vi "Autonomous Independent.vi"() -> ()   [LabVIEW 2017]
doc: "This VI is called when autonomous begins, and will automatically be terminated when autonomous ends. You can carry out timed or sensor driven robot movement independently without needing to return to the caller."
uses:
  2017_Steamworks/Programming_Team/Competition/Worlds/Labview/Global 2.vi
  MotionProfiling/FRC_Talon_Motion_Profiles_LV-master/Motion_Profiler_Class/Motion_Profiler_Class-323eb47bd4286328f3a3e236ed86bebf76c73fb1/MotionProfiles.lvclass
  <vilib>/Rock Robotics/Network Tables/NT Write Numeric Array.vi
  <vilib>/Rock Robotics/Network Tables/NT Read Number.vi
  <vilib>/Rock Robotics/Network Tables/NT Read String.vi
panel:
  out "Left Motor":T1(graph)
  out "Right Motor":T1(graph)
  out "Left Throttle":dbl
  out "Left Is Under Run":bool
  out "Left Bottom Buf Count":i32
  out "Right Throttle":dbl
  out "Right Is Under Run":bool
  out "Right Bottom Buf Count":i32
  out "Auto Mode":dbl
  out "Elapsed Time (s) 2":dbl=0.28672027587890625 caption="Elapsed Time (s)"
  out "Time has Elapsed 2":bool=TRUE caption="Time has Elapsed"
  out "Present (s) 2":dbl=3576229234.751028 caption="Present (s)"
  in  "Auton_Modes":T2(array[cluster])=[{"Actions"=[{"Effort"=0.55, "Duration"=3.5, "Action"=enum."Nothing", "Encoder"=0.0, "Condition"=FALSE}, {"Effort"=0.0, "Duration"=0.0, "Action"=enum."Nothing", "Encoder"=0.0, "Condition"=FALSE}]}, {"Actions"=[{"Effort"=0.0, "Duration"=0.1, "Action"=enum."Drive Encoder Reset", "Encoder"=0.0, "Condition"=FALSE}, {"Effort"=0.0, "Duration"=0.1, "Action"=enum."Gyro Reset", "Encoder"=0.0, "Condition"=FALSE}, {"Effort"=0.11, "Duration"=4.0, "Action"=enum."Drive", "Encoder"=72.0, "Condition"=FALSE}, {"Effort"=0.15, "Duration"=0.1, "Action"=enum."Turn", "Encoder"=-55.0, "Condition"=FALSE}, {"Effort"=0.0, "Duration"=0.1, "Action"=enum."Gyro Reset", "Encoder"=0.0, "Condition"=FALSE}, {"Effort"=0.0, "Duration"=0.1, "Action"=enum."Drive Encoder Reset", "Encoder"=0.0, "Condition"=FALSE}, {"Effort"=0.11, "Duration"=4.0, "Action"=enum."Drive", "Encoder"=66.0, "Condition"=FALSE}, {"Effort"=1.0, "Duration"=0.25, "Action"=enum."Gear0", "Encoder"=0.0, "Condition"=FALSE}, {"Effort"=0.0, "Duration"=0.1, "Action"=enum."Drive Encoder Reset", "Encoder"=0.0, "Condition"=FALSE}, {"Effort"=0.11, "Duration"=3.0, "Action"=enum."Drive", "Encoder"=-36.0, "Condition"=TRUE}, {"Effort"=0.08, "Duration"=0.0, "Action"=enum."Turn", "Encoder"=15.5, "Condition"=TRUE}, {"Effort"=0.0, "Duration"=10.0, "Action"=enum."Shoot", "Encoder"=0.0, "Condition"=FALSE}, {"Effort"=0.0, "Duration"=0.5, "Action"=enum."Nothing", "Encoder"=0.0, "Condition"=FALSE}, {"Effort"=0.0, "Duration"=5.0, "Action"=enum."Nothing", "Encoder"=-94.0, "Condition"=TRUE}]}, {"Actions"=[{"Effort"=0.0, "Duration"=0.1, "Action"=enum."Drive Encoder Reset", "Encoder"=0.0, "Condition"=FALSE}, {"Effort"=0.0, "Duration"=0.1, "Action"=enum."Gyro Reset", "Encoder"=0.0, "Condition"=FALSE}, {"Effort"=0.11, "Duration"=4.0, "Action"=enum."Drive", "Encoder"=76.0, "Condition"=FALSE}, {"Effort"=1.0, "Duration"=0.5, "Action"=enum."Gear0", "Encoder"=0.0, "Condition"=FALSE}, {"Effort"=1.0, "Duration"=0.0, "Action"=enum."Nothing", "Encoder"=0.0, "Condition"=FALSE}, {"Effort"=1.0, "Duration"=0.0, "Action"=enum."Nothing", "Encoder"=0.0, "Condition"=FALSE}, {"Effort"=0.0, "Duration"=0.0, "Action"=enum."Drive Encoder Reset", "Encoder"=0.0, "Condition"=FALSE}, {"Effort"=0.0, "Duration"=0.0, "Action"=enum."Nothing", "Encoder"=0.0, "Condition"=FALSE}, {"Effort"=0.0, "Duration"=0.0, "Action"=enum."Nothing", "Encoder"=0.0, "Condition"=FALSE}, {"Effort"=0.0, "Duration"=10000.0, "Action"=enum."Drive", "Encoder"=-24.0, "Condition"=FALSE}, {"Effort"=0.0, "Duration"=0.0, "Action"=enum."Drive Encoder Reset", "Encoder"=0.0, "Condition"=FALSE}, {"Effort"=-0.4, "Duration"=5.0, "Action"=enum."Nothing", "Encoder"=70.0, "Condition"=FALSE}]}, {"Actions"=[{"Effort"=0.0, "Duration"=0.1, "Action"=enum."Drive Encoder Reset", "Encoder"=6.462, "Condition"=FALSE}, {"Effort"=0.0, "Duration"=0.1, "Action"=enum."Gyro Reset", "Encoder"=0.0, "Condition"=FALSE}, {"Effort"=0.0, "Duration"=1.0, "Action"=enum."Drive", "Encoder"=60.0, "Condition"=FALSE}, {"Effort"=0.15, "Duration"=0.1, "Action"=enum."Turn", "Encoder"=55.0, "Condition"=FALSE}, {"Effort"=0.0, "Duration"=0.1, "Action"=enum."Gyro Reset", "Encoder"=0.0, "Condition"=FALSE}, {"Effort"=-0.25, "Duration"=0.0, "Action"=enum."Drive Encoder Reset", "Encoder"=7.5, "Condition"=FALSE}, {"Effort"=0.0, "Duration"=4.0, "Action"=enum."Drive", "Encoder"=76.0, "Condition"=FALSE}, {"Effort"=1.0, "Duration"=0.25, "Action"=enum."Gear0", "Encoder"=0.0, "Condition"=FALSE}, {"Effort"=0.0, "Duration"=0.1, "Action"=enum."Drive Encoder Reset", "Encoder"=0.0, "Condition"=FALSE}, {"Effort"=0.0, "Duration"=3.0, "Action"=enum."Drive", "Encoder"=-36.0, "Condition"=FALSE}, {"Effort"=0.08, "Duration"=0.0, "Action"=enum."Turn", "Encoder"=-60.0, "Condition"=FALSE}, {"Effort"=0.0, "Duration"=0.1, "Action"=enum."Gyro Reset", "Encoder"=0.0, "Condition"=FALSE}, {"Effort"=0.0, "Duration"=0.5, "Action"=enum."Drive Encoder Reset", "Encoder"=0.0, "Condition"=FALSE}, {"Effort"=0.0, "Duration"=5.0, "Action"=enum."Drive", "Encoder"=30.0, "Condition"=TRUE}]}, {"Actions"=[{"Effort"=0.0, "Duration"=0.1, "Action"=enum."Drive Encoder Reset", "Encoder"=6.462, "Condition"=FALSE}, {"Effort"=0.0, "Duration"=0.1, "Action"=enum."Gyro Reset", "Encoder"=0.0, "Condition"=FALSE}, {"Effort"=0.0, "Duration"=1.0, "Action"=enum."Drive", "Encoder"=60.0, "Condition"=FALSE}, {"Effort"=0.15, "Duration"=0.1, "Action"=enum."Turn", "Encoder"=-55.0, "Condition"=FALSE}, {"Effort"=0.0, "Duration"=0.1, "Action"=enum."Gyro Reset", "Encoder"=0.0, "Condition"=FALSE}, {"Effort"=-0.25, "Duration"=0.0, "Action"=enum."Drive Encoder Reset", "Encoder"=7.5, "Condition"=FALSE}, {"Effort"=0.0, "Duration"=4.0, "Action"=enum."Drive", "Encoder"=76.0, "Condition"=FALSE}, {"Effort"=1.0, "Duration"=0.25, "Action"=enum."Gear0", "Encoder"=0.0, "Condition"=FALSE}, {"Effort"=0.0, "Duration"=0.1, "Action"=enum."Drive Encoder Reset", "Encoder"=0.0, "Condition"=FALSE}, {"Effort"=0.0, "Duration"=3.0, "Action"=enum."Drive", "Encoder"=-36.0, "Condition"=FALSE}, {"Effort"=0.08, "Duration"=0.0, "Action"=enum."Turn", "Encoder"=60.0, "Condition"=FALSE}, {"Effort"=0.0, "Duration"=0.1, "Action"=enum."Gyro Reset", "Encoder"=0.0, "Condition"=FALSE}, {"Effort"=0.0, "Duration"=0.5, "Action"=enum."Drive Encoder Reset", "Encoder"=0.0, "Condition"=FALSE}, {"Effort"=0.0, "Duration"=5.0, "Action"=enum."Drive", "Encoder"=30.0, "Condition"=TRUE}]}, {"Actions"=[{"Effort"=0.0, "Duration"=0.1, "Action"=enum."Drive Encoder Reset", "Encoder"=0.0, "Condition"=FALSE}, {"Effort"=0.0, "Duration"=0.1, "Action"=enum."Gyro Reset", "Encoder"=0.0, "Condition"=FALSE}, {"Effort"=0.11, "Duration"=4.0, "Action"=enum."Drive", "Encoder"=72.0, "Condition"=FALSE}, {"Effort"=0.08, "Duration"=0.1, "Action"=enum."Turn", "Encoder"=58.0, "Condition"=FALSE}, {"Effort"=0.0, "Duration"=0.1, "Action"=enum."Gyro Reset", "Encoder"=0.0, "Condition"=FALSE}, {"Effort"=0.0, "Duration"=0.1, "Action"=enum."Drive Encoder Reset", "Encoder"=0.0, "Condition"=FALSE}, {"Effort"=0.11, "Duration"=4.0, "Action"=enum."Drive", "Encoder"=72.0, "Condition"=FALSE}, {"Effort"=1.0, "Duration"=0.25, "Action"=enum."Gear0", "Encoder"=0.0, "Condition"=FALSE}, {"Effort"=0.0, "Duration"=0.1, "Action"=enum."Drive Encoder Reset", "Encoder"=3.0, "Condition"=FALSE}, {"Effort"=0.11, "Duration"=3.0, "Action"=enum."Drive", "Encoder"=-36.0, "Condition"=FALSE}, {"Effort"=0.08, "Duration"=0.0, "Action"=enum."Turn", "Encoder"=-15.5, "Condition"=FALSE}, {"Effort"=0.0, "Duration"=10.0, "Action"=enum."Nothing", "Encoder"=0.0, "Condition"=FALSE}, {"Effort"=0.0, "Duration"=0.5, "Action"=enum."Nothing", "Encoder"=0.0, "Condition"=FALSE}, {"Effort"=0.11, "Duration"=0.0, "Action"=enum."Nothing", "Encoder"=-94.0, "Condition"=FALSE}, {"Effort"=0.0, "Duration"=10.0, "Action"=enum."Nothing", "Encoder"=0.0, "Condition"=FALSE}]}, {"Actions"=[{"Effort"=0.0, "Duration"=0.1, "Action"=enum."Drive Encoder Reset", "Encoder"=0.0, "Condition"=FALSE}, {"Effort"=0.0, "Duration"=0.1, "Action"=enum."Gyro Reset", "Encoder"=0.0, "Condition"=FALSE}, {"Effort"=0.2, "Duration"=5.0, "Action"=enum."Drive", "Encoder"=110.0, "Condition"=FALSE}, {"Effort"=0.75, "Duration"=1.0, "Action"=enum."Nothing", "Encoder"=0.0, "Condition"=FALSE}, {"Effort"=0.0, "Duration"=1.0, "Action"=enum."Nothing", "Encoder"=0.0, "Condition"=FALSE}, {"Effort"=0.0, "Duration"=0.0, "Action"=enum."Nothing", "Encoder"=0.0, "Condition"=FALSE}]}, {"Actions"=[{"Effort"=0.0, "Duration"=0.1, "Action"=enum."Drive Encoder Reset", "Encoder"=0.0, "Condition"=FALSE}, {"Effort"=0.0, "Duration"=0.1, "Action"=enum."Gyro Reset", "Encoder"=0.0, "Condition"=FALSE}, {"Effort"=0.3, "Duration"=0.0, "Action"=enum."Drive", "Encoder"=24.0, "Condition"=FALSE}, {"Effort"=0.3, "Duration"=3.0, "Action"=enum."Nothing", "Encoder"=0.0, "Condition"=FALSE}, {"Effort"=0.3, "Duration"=2.0, "Action"=enum."Vision Correction", "Encoder"=30.0, "Condition"=FALSE}, {"Effort"=0.2, "Duration"=1.0, "Action"=enum."Drive", "Encoder"=18.5, "Condition"=TRUE}, {"Effort"=1.0, "Duration"=0.0, "Action"=enum."Gear0", "Encoder"=0.0, "Condition"=FALSE}, {"Effort"=-0.2, "Duration"=1.3, "Action"=enum."Drive", "Encoder"=30.0, "Condition"=TRUE}, {"Effort"=0.0, "Duration"=3.0, "Action"=enum."Nothing", "Encoder"=0.0, "Condition"=FALSE}, {"Effort"=0.03, "Duration"=0.0, "Action"=enum."Turn", "Encoder"=0.0, "Condition"=FALSE}, {"Effort"=0.0, "Duration"=0.0, "Action"=enum."Drive", "Encoder"=0.0, "Condition"=FALSE}]}, {"Actions"=[{"Effort"=0.0, "Duration"=0.0, "Action"=enum."Nothing", "Encoder"=0.0, "Condition"=FALSE}]}, {"Actions"=[{"Effort"=0.0, "Duration"=2.5, "Action"=enum."Shoot", "Encoder"=0.0, "Condition"=FALSE}, {"Effort"=0.0, "Duration"=5.0, "Action"=enum."Index", "Encoder"=0.0, "Condition"=FALSE}, {"Effort"=0.25, "Duration"=3.5, "Action"=enum."Nothing", "Encoder"=88.0, "Condition"=FALSE}, {"Effort"=1.0, "Duration"=1.0, "Action"=enum."Nothing", "Encoder"=0.0, "Condition"=FALSE}, {"Effort"=1.0, "Duration"=1.0, "Action"=enum."Nothing", "Encoder"=0.0, "Condition"=FALSE}, {"Effort"=1.0, "Duration"=0.5, "Action"=enum."Nothing", "Encoder"=0.0, "Condition"=FALSE}, {"Effort"=0.0, "Duration"=0.0, "Action"=enum."Nothing", "Encoder"=0.0, "Condition"=FALSE}, {"Effort"=-0.25, "Duration"=0.0, "Action"=enum."Nothing", "Encoder"=3.0, "Condition"=FALSE}, {"Effort"=0.0, "Duration"=0.0, "Action"=enum."Nothing", "Encoder"=0.0, "Condition"=FALSE}, {"Effort"=0.25, "Duration"=0.0, "Action"=enum."Nothing", "Encoder"=24.0, "Condition"=FALSE}, {"Effort"=0.0, "Duration"=0.0, "Action"=enum."Nothing", "Encoder"=0.0, "Condition"=FALSE}, {"Effort"=-0.25, "Duration"=0.0, "Action"=enum."Nothing", "Encoder"=12.0, "Condition"=FALSE}]}, {"Actions"=[{"Effort"=0.0, "Duration"=0.1, "Action"=enum."Drive Encoder Reset", "Encoder"=0.0, "Condition"=FALSE}, {"Effort"=0.0, "Duration"=1.0, "Action"=enum."Gyro Reset", "Encoder"=0.0, "Condition"=FALSE}, {"Effort"=0.3, "Duration"=1.4, "Action"=enum."Drive", "Encoder"=88.0, "Condition"=FALSE}, {"Effort"=0.3, "Duration"=3.0, "Action"=enum."Turn", "Encoder"=2.0, "Condition"=FALSE}, {"Effort"=1.0, "Duration"=1.0, "Action"=enum."Nothing", "Encoder"=0.0, "Condition"=FALSE}, {"Effort"=1.0, "Duration"=1.0, "Action"=enum."Nothing", "Encoder"=0.0, "Condition"=FALSE}, {"Effort"=0.0, "Duration"=0.0, "Action"=enum."Nothing", "Encoder"=0.0, "Condition"=FALSE}, {"Effort"=-0.25, "Duration"=0.0, "Action"=enum."Nothing", "Encoder"=3.0, "Condition"=FALSE}, {"Effort"=0.0, "Duration"=0.0, "Action"=enum."Nothing", "Encoder"=0.0, "Condition"=FALSE}, {"Effort"=0.25, "Duration"=0.0, "Action"=enum."Nothing", "Encoder"=24.0, "Condition"=FALSE}, {"Effort"=0.0, "Duration"=0.0, "Action"=enum."Nothing", "Encoder"=0.0, "Condition"=FALSE}, {"Effort"=-0.25, "Duration"=0.0, "Action"=enum."Nothing", "Encoder"=12.0, "Condition"=FALSE}]}, {"Actions"=[{"Effort"=0.0, "Duration"=1.0, "Action"=enum."Drive Encoder Reset", "Encoder"=0.0, "Condition"=FALSE}, {"Effort"=0.0, "Duration"=1.0, "Action"=enum."Shoot", "Encoder"=0.0, "Condition"=FALSE}, {"Effort"=0.25, "Duration"=5.0, "Action"=enum."Index", "Encoder"=88.0, "Condition"=FALSE}, {"Effort"=1.0, "Duration"=1.0, "Action"=enum."Nothing", "Encoder"=0.0, "Condition"=FALSE}, {"Effort"=1.0, "Duration"=1.0, "Action"=enum."Nothing", "Encoder"=0.0, "Condition"=FALSE}, {"Effort"=1.0, "Duration"=0.5, "Action"=enum."Nothing", "Encoder"=0.0, "Condition"=FALSE}, {"Effort"=0.0, "Duration"=0.0, "Action"=enum."Nothing", "Encoder"=0.0, "Condition"=FALSE}, {"Effort"=-0.25, "Duration"=0.0, "Action"=enum."Nothing", "Encoder"=3.0, "Condition"=FALSE}, {"Effort"=0.0, "Duration"=0.0, "Action"=enum."Nothing", "Encoder"=0.0, "Condition"=FALSE}, {"Effort"=0.25, "Duration"=0.0, "Action"=enum."Nothing", "Encoder"=24.0, "Condition"=FALSE}, {"Effort"=0.0, "Duration"=0.0, "Action"=enum."Nothing", "Encoder"=0.0, "Condition"=FALSE}, {"Effort"=-0.25, "Duration"=0.0, "Action"=enum."Nothing", "Encoder"=12.0, "Condition"=FALSE}]}, {"Actions"=[{"Effort"=0.0, "Duration"=0.1, "Action"=enum."Drive Encoder Reset", "Encoder"=0.0, "Condition"=FALSE}, {"Effort"=0.0, "Duration"=1.0, "Action"=enum."Gyro Reset", "Encoder"=0.0, "Condition"=FALSE}, {"Effort"=0.0, "Duration"=20.0, "Action"=enum."Drive", "Encoder"=60.0, "Condition"=FALSE}, {"Effort"=0.3, "Duration"=4.0, "Action"=enum."Nothing", "Encoder"=0.0, "Condition"=FALSE}, {"Effort"=1.0, "Duration"=1.0, "Action"=enum."Nothing", "Encoder"=0.0, "Condition"=FALSE}, {"Effort"=1.0, "Duration"=0.5, "Action"=enum."Nothing", "Encoder"=0.0, "Condition"=FALSE}, {"Effort"=0.0, "Duration"=0.0, "Action"=enum."Nothing", "Encoder"=0.0, "Condition"=FALSE}, {"Effort"=0.3, "Duration"=0.5, "Action"=enum."Nothing", "Encoder"=24.0, "Condition"=TRUE}, {"Effort"=0.0, "Duration"=0.0, "Action"=enum."Nothing", "Encoder"=0.0, "Condition"=FALSE}, {"Effort"=-0.2, "Duration"=2.0, "Action"=enum."Nothing", "Encoder"=24.0, "Condition"=TRUE}, {"Effort"=0.0, "Duration"=0.0, "Action"=enum."Nothing", "Encoder"=0.0, "Condition"=FALSE}, {"Effort"=-0.25, "Duration"=0.0, "Action"=enum."Nothing", "Encoder"=12.0, "Condition"=FALSE}]}, {"Actions"=[{"Effort"=0.0, "Duration"=0.1, "Action"=enum."Drive Encoder Reset", "Encoder"=0.0, "Condition"=FALSE}, {"Effort"=0.0, "Duration"=0.1, "Action"=enum."Gyro Reset", "Encoder"=0.0, "Condition"=FALSE}, {"Effort"=0.0, "Duration"=4.0, "Action"=enum."Nothing", "Encoder"=4.0, "Condition"=FALSE}, {"Effort"=0.3, "Duration"=0.1, "Action"=enum."Vision Correction", "Encoder"=24.0, "Condition"=FALSE}, {"Effort"=0.0, "Duration"=0.1, "Action"=enum."Nothing", "Encoder"=0.0, "Condition"=FALSE}, {"Effort"=0.3, "Duration"=4.0, "Action"=enum."Nothing", "Encoder"=68.17, "Condition"=FALSE}, {"Effort"=1.0, "Duration"=0.25, "Action"=enum."Nothing", "Encoder"=0.0, "Condition"=FALSE}, {"Effort"=0.0, "Duration"=0.0, "Action"=enum."Nothing", "Encoder"=3.0, "Condition"=FALSE}, {"Effort"=-0.3, "Duration"=3.0, "Action"=enum."Nothing", "Encoder"=36.0, "Condition"=FALSE}, {"Effort"=0.15, "Duration"=0.0, "Action"=enum."Nothing", "Encoder"=31.5, "Condition"=FALSE}, {"Effort"=0.0, "Duration"=0.1, "Action"=enum."Nothing", "Encoder"=0.0, "Condition"=FALSE}]}]
  # "Be sure to right-click and choose Data Operations>>Make Current Value default if you want to save the array values with the VI"
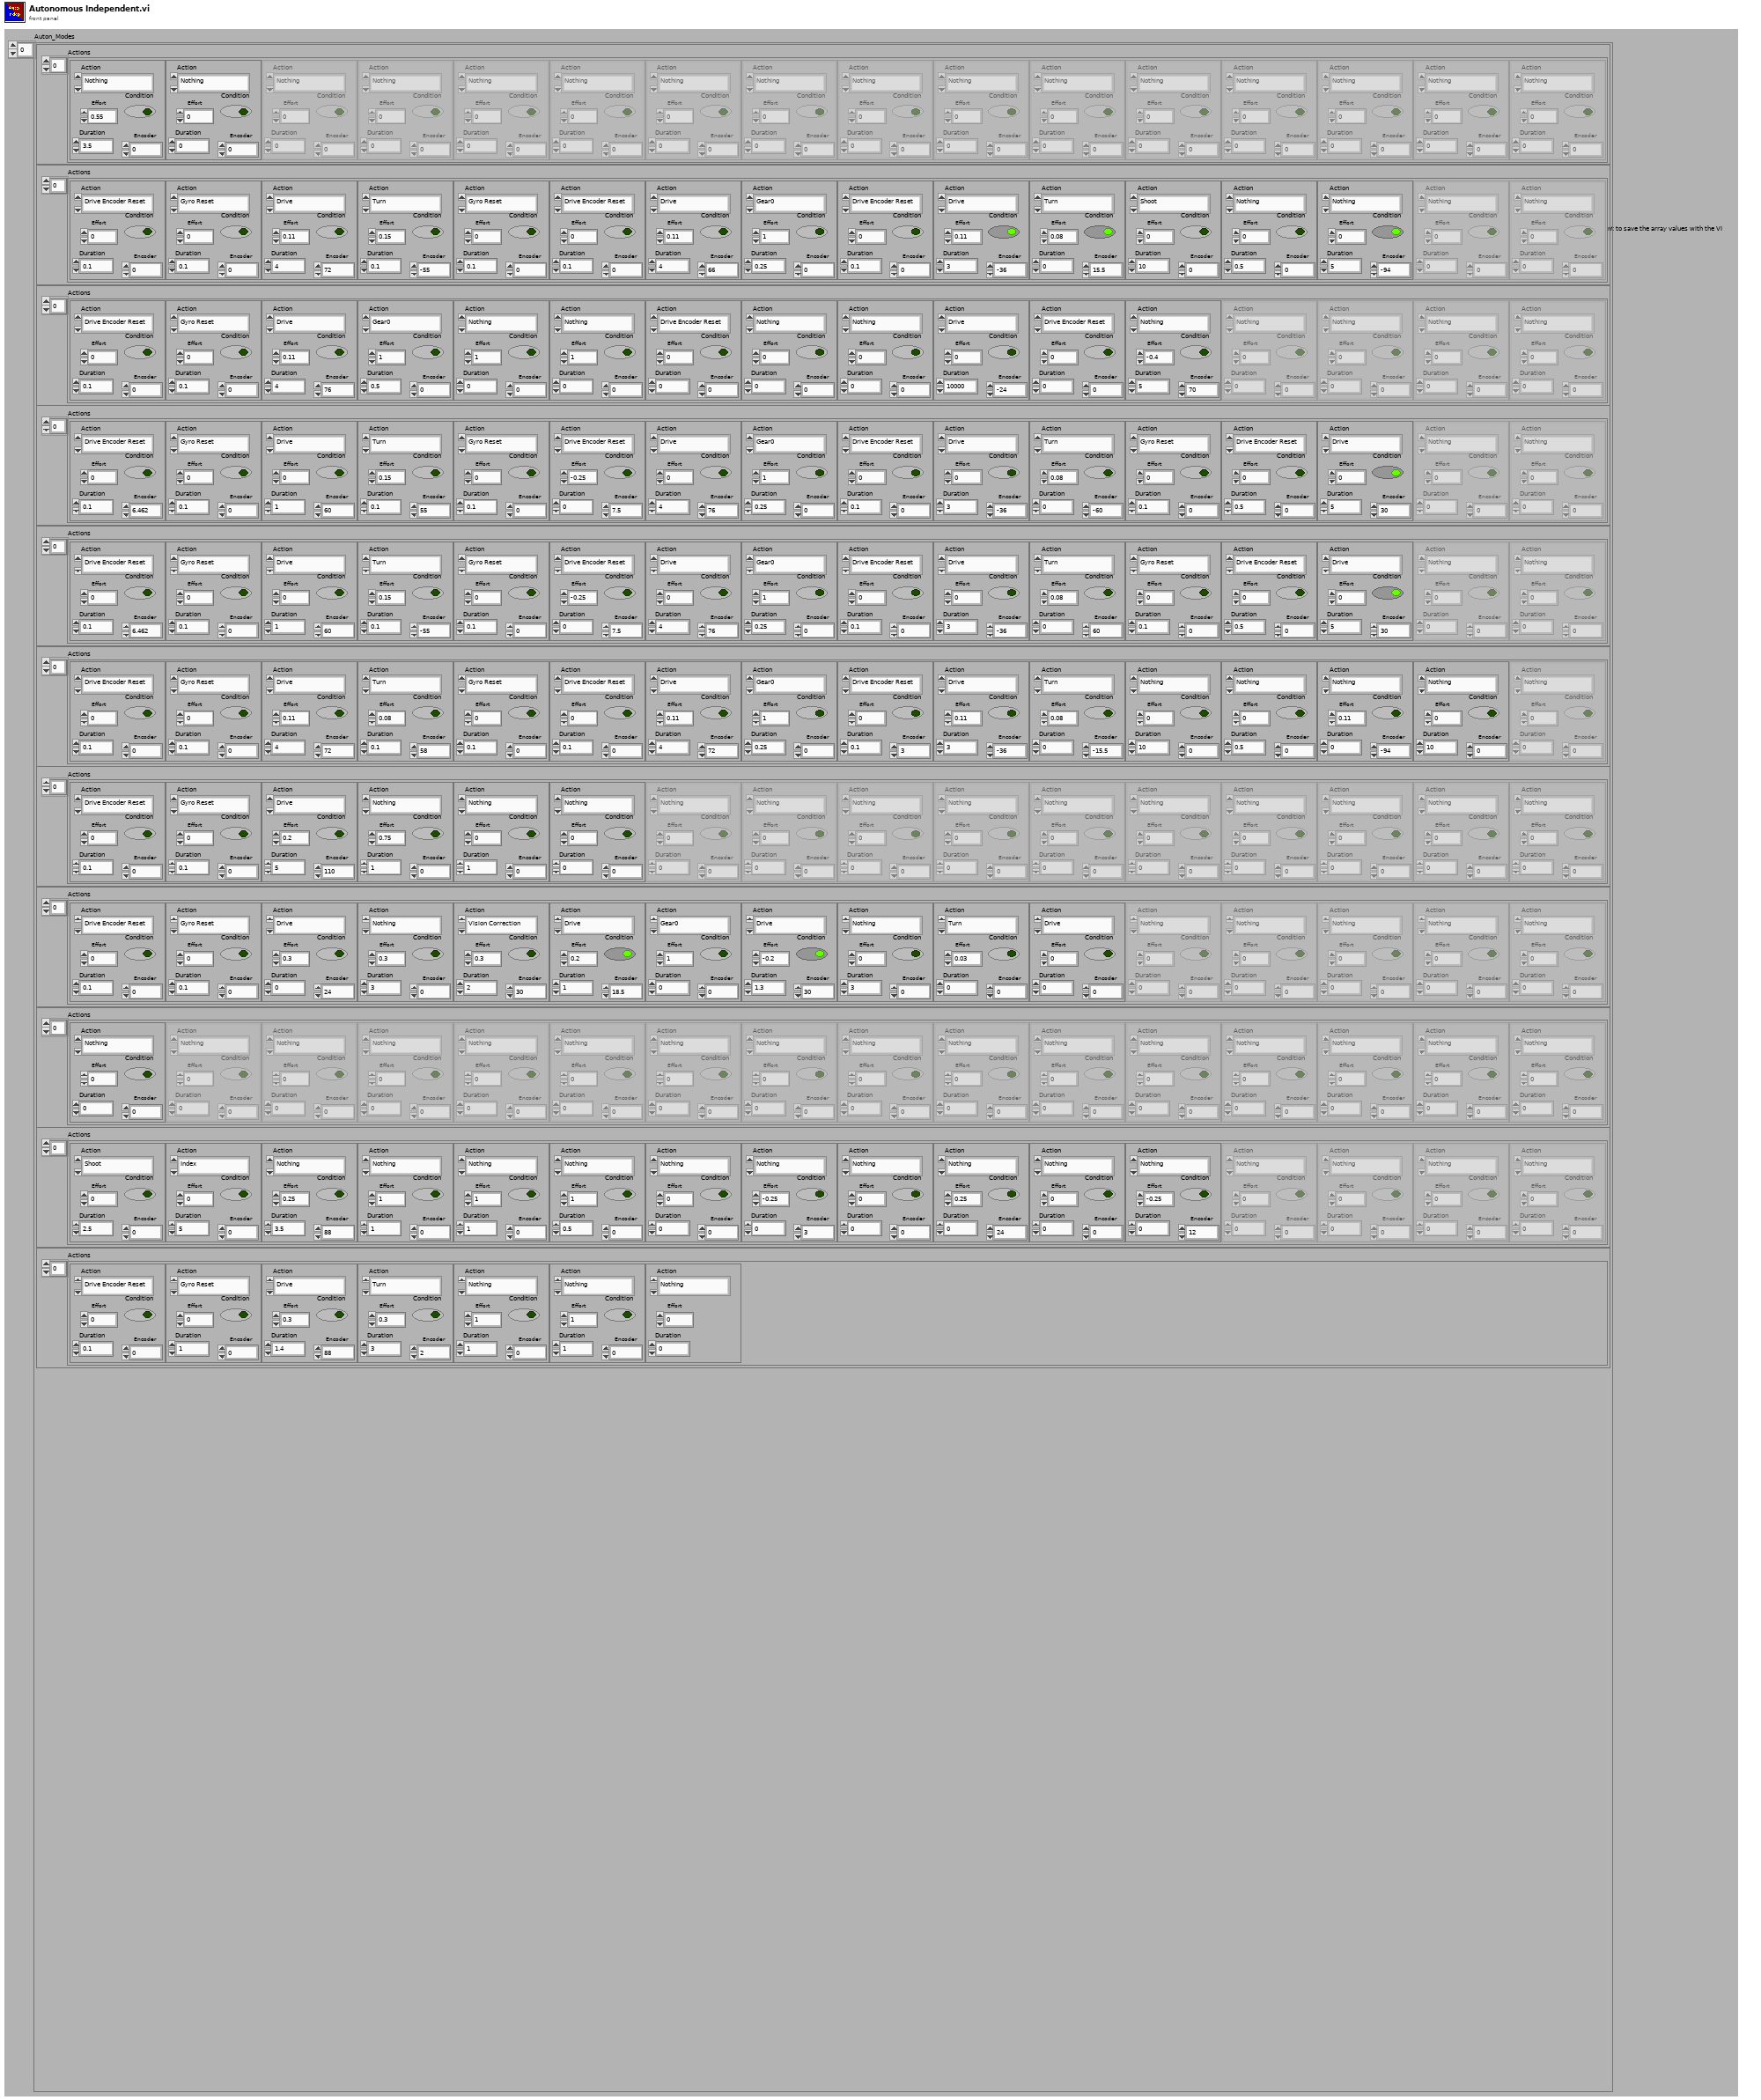
[diagram p1: front panel]
types:
  T1 = cluster{"Set_Vel_(u/100ms)":i32, "Act_Vel_(u/100ms)":i32, "Set_Pos_(u)":i32, "Act_Pos(u)":i32}
  T2 = cluster{"Actions":cluster{"Effort":dbl, "Duration":dbl, "Action":enum16{"Nothing", "Drive", "Vision Correction", "Turn", "Gear0", "Gear1", "Climb", "Intake", "Index", "Shoot", "Test", "Drive Encoder Reset", "Gyro Reset"}, "Encoder":dbl, "Condition":bool}[]}[]
  T3 = typedef "WPI_JoystickDevRef.ctl" = cluster{"Device":T4}
  T4 = typedef "WPI_JoystickDeviceEnum.ctl" = enum16{"USB 0", "USB 1", "USB 2", "USB 3", "USB 4", "USB 5"}
  T5 = cluster{"Actions":cluster{"Effort":dbl, "Duration":dbl, "Action":enum16{"Nothing", "Drive", "Vision Correction", "Turn", "Gear0", "Gear1", "Climb", "Intake", "Index", "Shoot", "Test", "Drive Encoder Reset", "Gyro Reset"}, "Encoder":dbl, "Condition":bool}[]}
  T6 = cluster{"Effort":dbl, "Duration":dbl, "Action":enum16{"Nothing", "Drive", "Vision Correction", "Turn", "Gear0", "Gear1", "Climb", "Intake", "Index", "Shoot", "Test", "Drive Encoder Reset", "Gyro Reset"}, "Encoder":dbl, "Condition":bool}[]
  T7 = typedef "WPI_MotorControlDeviceRef.ctl" = cluster{"DeviceStatus":errorcluster, "Type":T8, "PWM":cluster{"PWM Channel":T9, "DeadBand":T10}, "CAN":cluster{"Device Number":u8, "SetOutput VI Ref":variant, "GetOutput VI Ref":variant, "Enable VI Ref":variant, "Disable VI Ref":variant, "Data":variant}, "Invert":bool, "DIO PWM":cluster{"PWM \"Enable\" Channel":T9, "DIOChannel":T11, "PWM Rate":dbl}}
  T8 = typedef "WPI_MotorControlType.ctl" = enum16{"PWM", "CAN", "DIO PWM"}
  T9 = typedef "FPGA_DIOPWMChannel.ctl" = enum8{"PWM 0", "PWM 1", "PWM 2", "PWM 3", "PWM 4", "PWM 5", "PWM 6", "PWM 7", "PWM 8", "PWM 9", "PWM MXP 0", "PWM MXP 1", "PWM MXP 2", "PWM MXP 3", "PWM MXP 4", "PWM MXP 5", "PWM MXP 6", "PWM MXP 7", "PWM MXP 8", "PWM MXP 9", "Invalid"}
  T10 = typedef "WPI_PWMDeadband.ctl" = cluster{"Name":string, "maxPositivePwm":i32, "minPositivePwm":i32, "centerPwm":i32, "maxNegativePwm":i32, "minNegativePwm":i32, "angularRange":u16}
  T11 = typedef "FPGA_DIOChannel.ctl" = enum8{"DIO 0", "DIO 1", "DIO 2", "DIO 3", "DIO 4", "DIO 5", "DIO 6", "DIO 7", "DIO 8", "DIO 9", "DIO MXP 0", "DIO MXP 1", "DIO MXP 2", "DIO MXP 3", "DIO MXP 4", "DIO MXP 5", "DIO MXP 6", "DIO MXP 7", "DIO MXP 8", "DIO MXP 9", "DIO MXP 10", "DIO MXP 11", "DIO MXP 12", "DIO MXP 13", "DIO MXP 14", "DIO MXP 15", "SPI Port CS1", "SPI Port CS2", "SPI Port CS3", "SPI Port MISO", "SPI Port MOSI", "Invalid"}
  T12 = enum16{"Nothing", "Drive", "Vision Correction", "Turn", "Gear0", "Gear1", "Climb", "Intake", "Index", "Shoot", "Test", "Drive Encoder Reset", "Gyro Reset"}
  T13 = typedef "MotionProfiles.lvclass/MotionProfile_MP_Class_Status.ctl" = cluster{"Motion Profile Status":cluster{"Top Buffer Remaining":i32, "Top Buffer Count":i32, "Bottom Buffer Count":i32, "Has Underrun?":bool, "Is Underrun?":bool, "Active Point Valid?":bool, "Is Last?":bool, "Profile Slot Select 0":i32, "Output Enable":i32, "Time Duration (ms)":i32, "Profile Slot Select 1":i32}, "TalonState":T14, "MP Is Done":bool, "MP Is Executing":bool, "Set_Vel_(u/100ms)":i32, "Set_Pos_(u)":i32, "Act_Vel_(u/100ms)":i32, "Act_Pos(u)":i32, "Throtle":dbl}
  T14 = typedef "MotionProfiles.lvclass/MotionProfile_TalonSetValueEnum.ctl" = enum16{"Disable", "Enable", "Hold"}
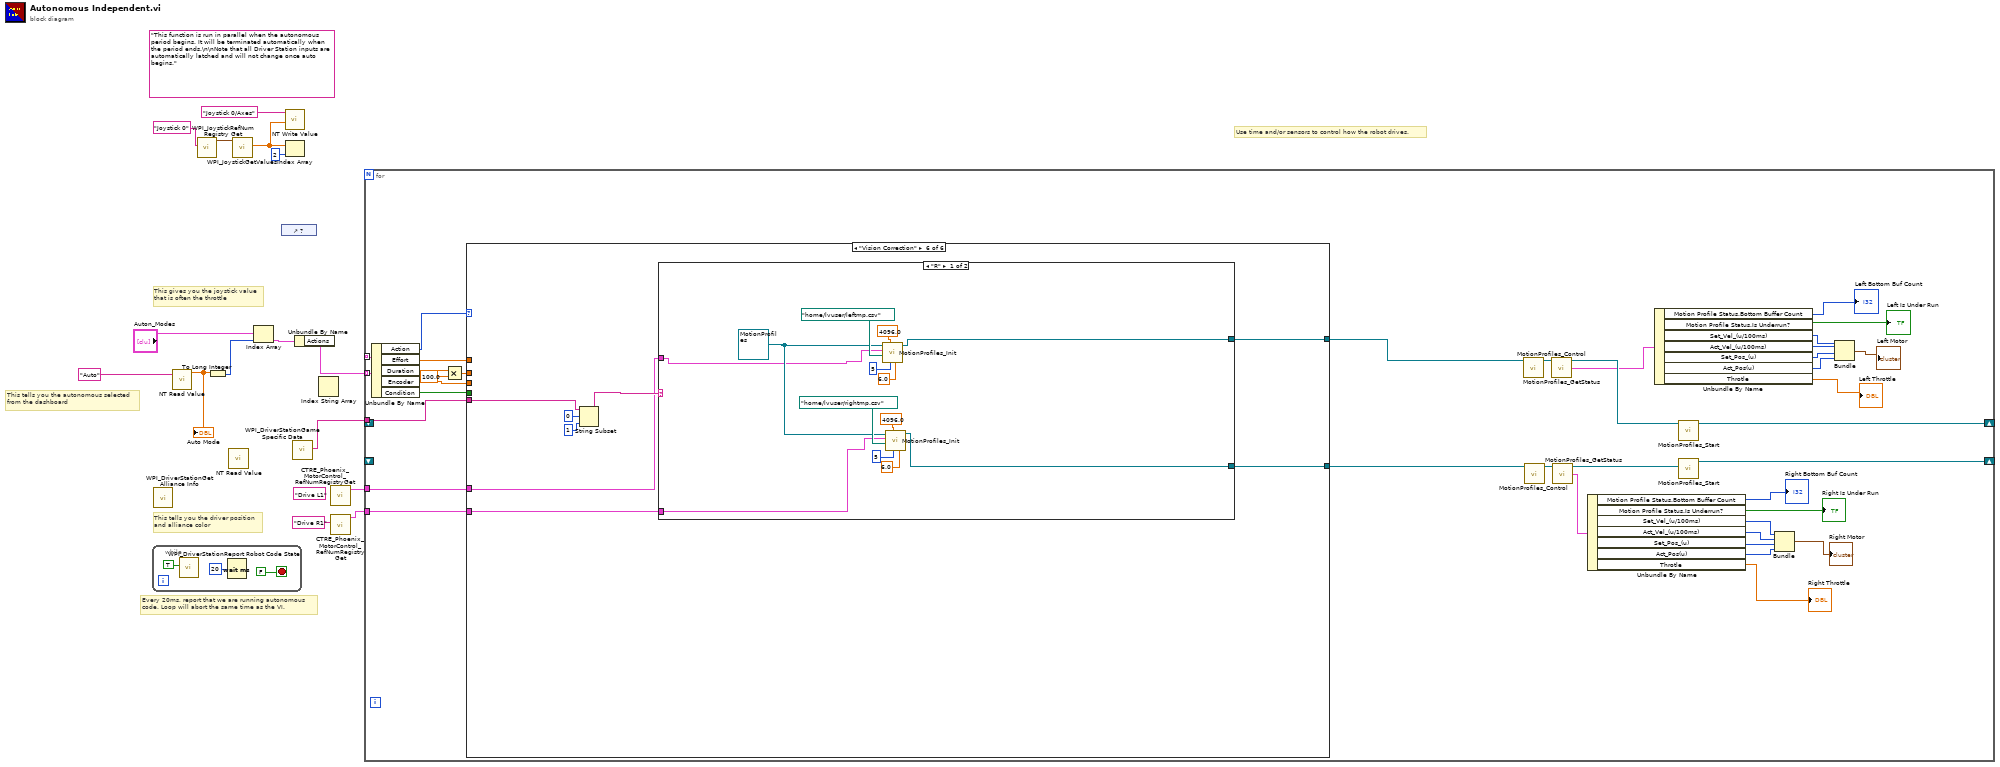
[diagram p0: block diagram]
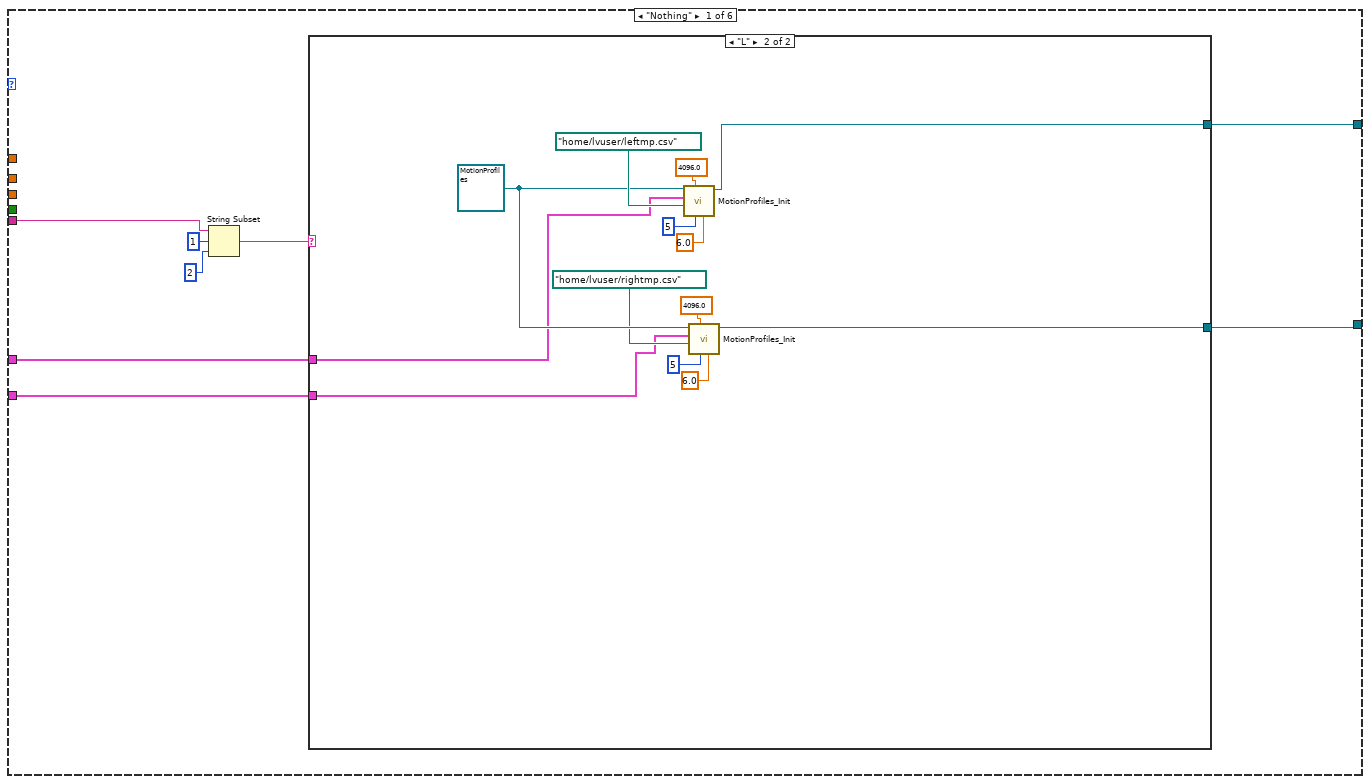
[diagram p2: hidden frame]
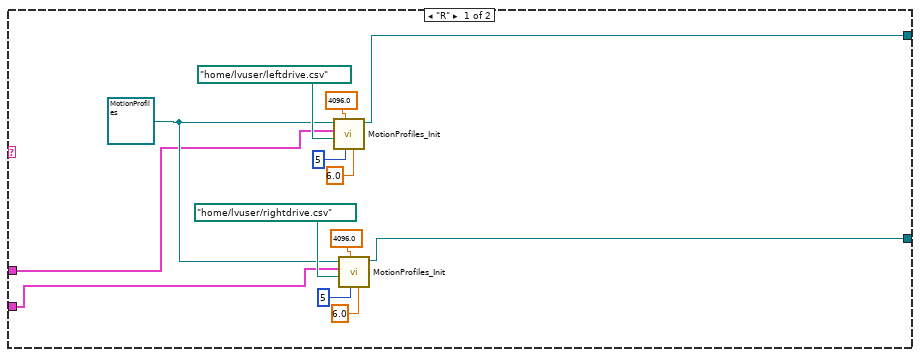
[diagram p3: hidden frame]
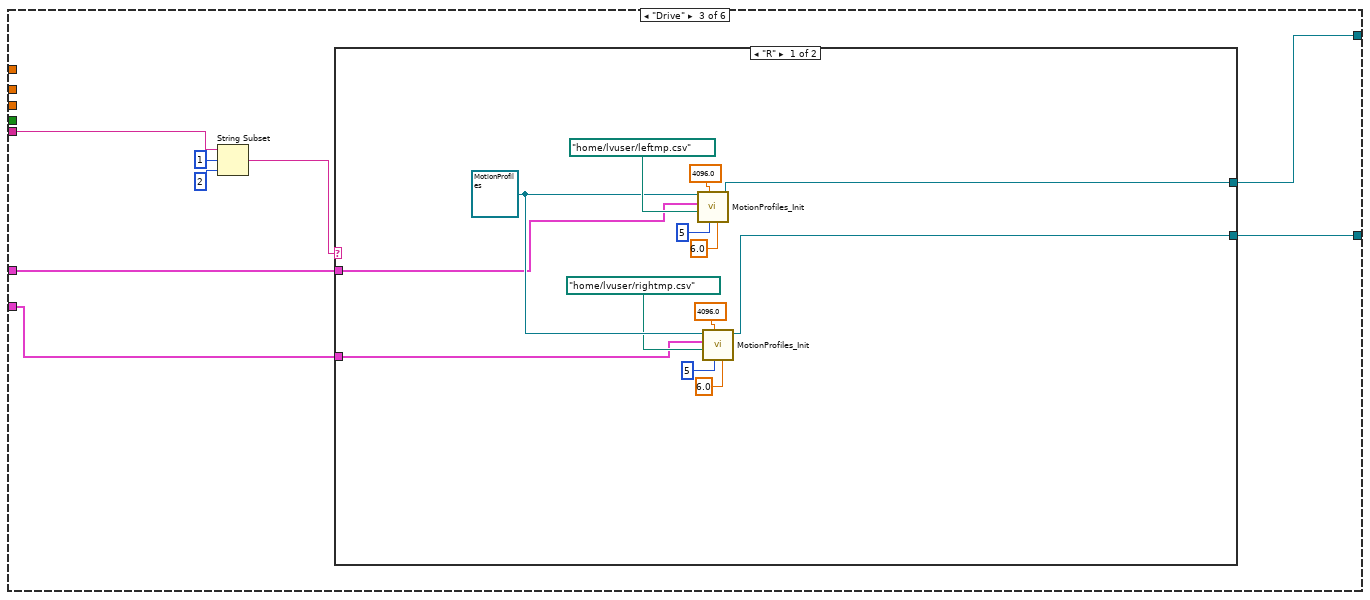
[diagram p5: hidden frame]
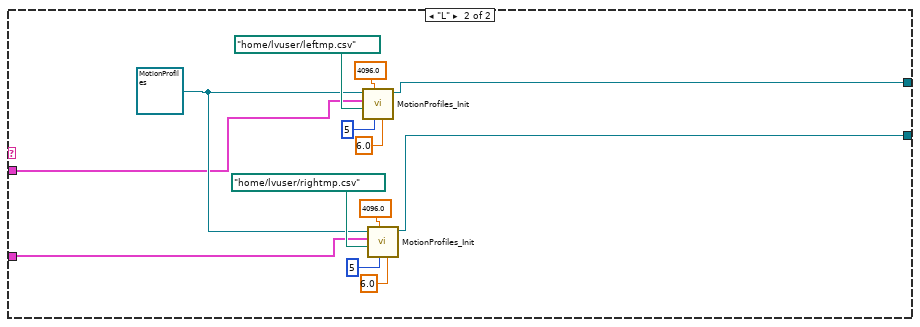
[diagram p6: hidden frame]
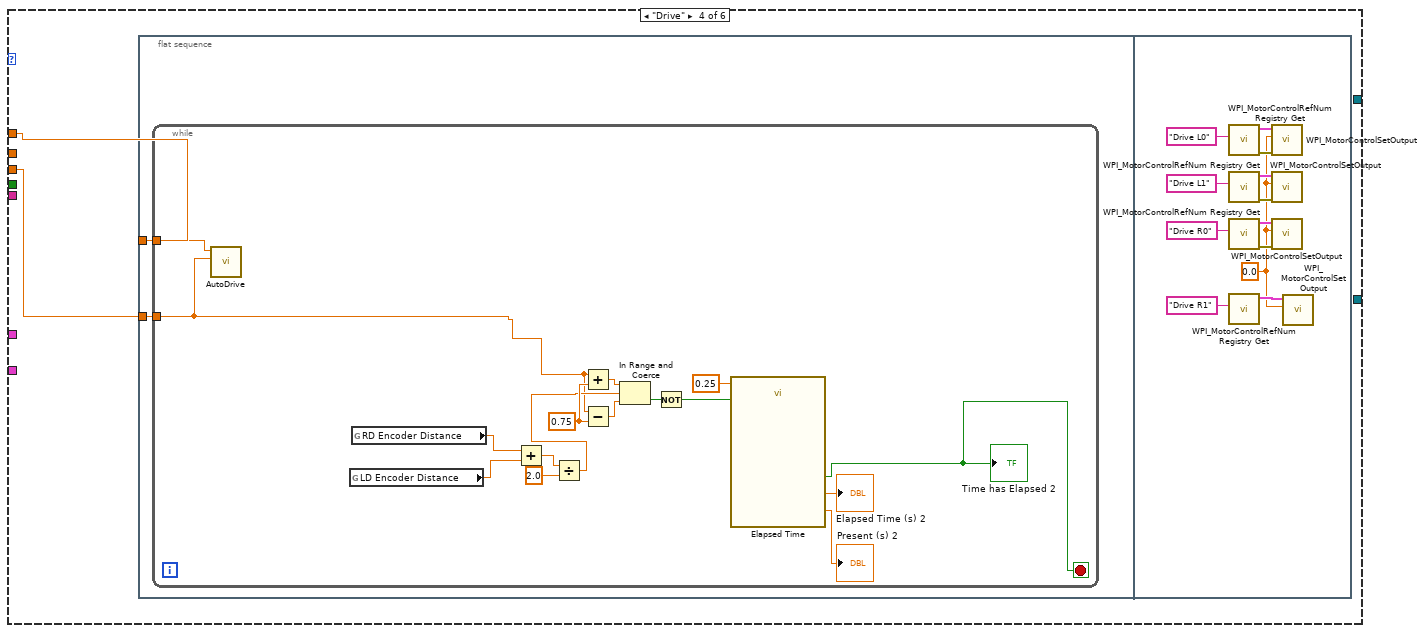
[diagram p7: hidden frame]
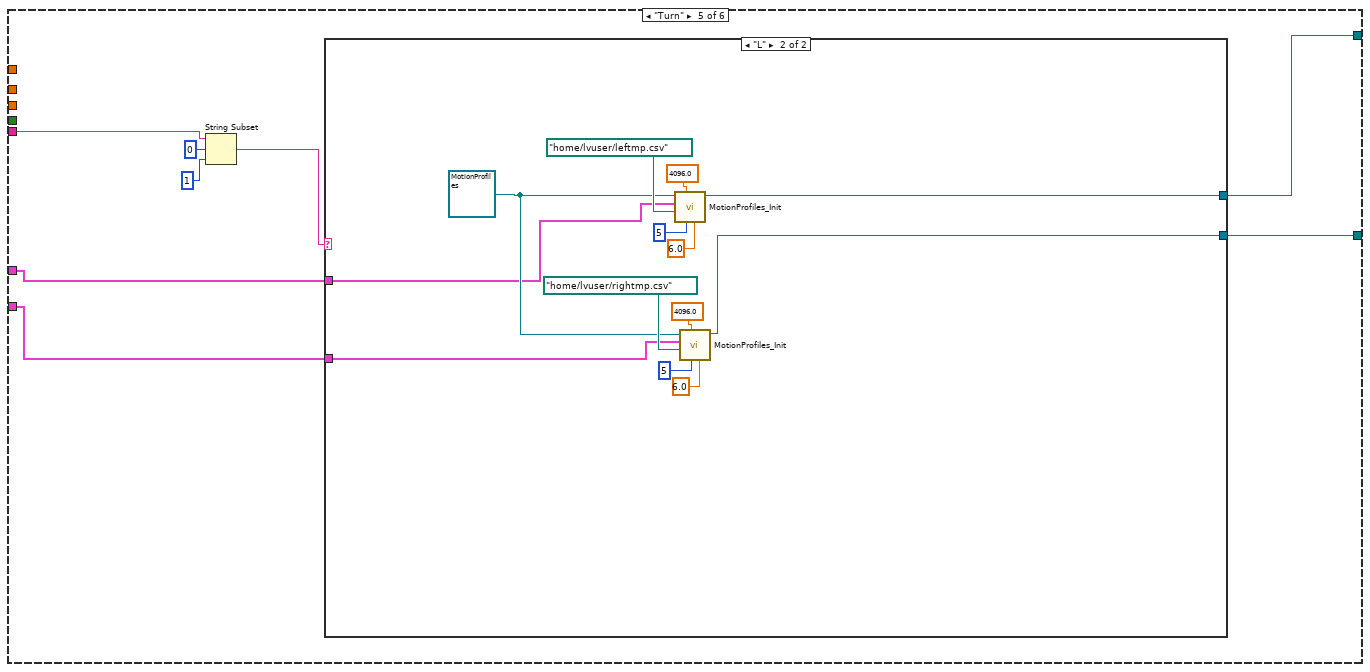
[diagram p8: hidden frame]
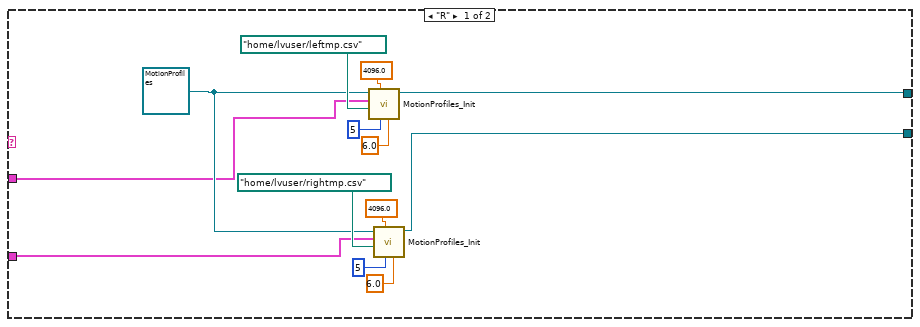
[diagram p9: hidden frame]
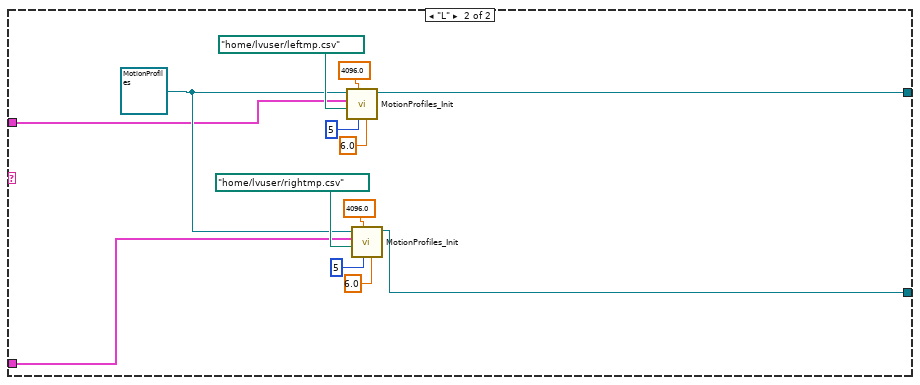
[diagram p10: hidden frame]
diagram:
  (unwired) "Drive L1" ("refnum name")
  (unwired) "This function is run in parallel when the autonomous period begins. It will be terminated automatically when the period ends.\n\nNote that all Driver Station inputs are automatically latched and will not change once auto begins."
  # "This tells you the autonomous selected\nfrom the dashboard"
  # "Every 20ms, report that we are running autonomous\ncode. Loop will abort the same time as the VI."
  # "This gives you the joystick value\nthat is often the throttle"
  # "Use time and/or sensors to control how the robot drives."
  # "This tells you the driver position\nand alliance color"
  n1 = while {
    stop <- FALSE stop-if-true
    n2 = call <vilib>:"WPI_DriverStationReport Robot Code State.vi"("Autonomous"=TRUE) -> ()  [unwired: 10 in, 1 out]
    n3 = Wait (ms)(milliseconds to wait=u32 20) -> ()  [unwired: 1 out]
  }
  n4 = call <vilib>:"WPI_DriverStationGet Alliance Info.vi"() -> ()  [unwired: 12 out]
  n5 = call-poly <vilib>:"NT Read Value.vi"("Name"="Auto") -> ("Numeric"=w9:dbl)  [unwired: 9 in, 1 out]
  "Auto Mode" <- w9
  n6 = call <vilib>:"WPI_JoystickRefNum Registry Get.vi"("refnum name"="Joystick 0") -> ("JoystickDevRef"=w14:T3)  [unwired: 1 in, 9 out]
  n7 = To Long Integer(number=w9) -> (32bit integer=w8:i32)
  n8 = call-poly <vilib>:"NT Read Value.vi"() -> ()  [unwired: 10 in, 2 out]
  n9 = call <vilib>:"WPI_JoystickGetValues.vi"("JoystickDevRef"=w14) -> ("Axes"=w11:dbl[])  [unwired: 6 in, 4 out]
  n10 = Index Array(array="Auton_Modes", index=w8) -> (element=w5:T5)
  n11 = control-ref of="?"() -> ()  [unwired: 1 out]
  n12 = call-poly <vilib>:"NT Write Value.vi"("Numeric Array"=w11, "Name"="Joystick 0/Axes") -> ()  [unwired: 9 in, 1 out]
  n13 = Index Array(array=w11, index=2) -> ()  [unwired: 1 out]
  n14 = call <vilib>:"WPI_DriverStationGame Specific Data.vi"() -> ("Game Specific Data"=w6:string)  [unwired: 11 in]
  n15 = Unbundle By Name(w5) -> ("Actions"=w4:T6)
  n16 = Index String Array() -> ()  [unwired: 3 in, 1 out]
  n17 = call <vilib>:"CTRE_Phoenix_MotorControl_RefNumRegistryGet.vi"("refnum name"="Drive R1") -> ("PhoenixMotorControlDevRef"=w1:T7)  [unwired: 9 in, 1 out]
  n18 = call <vilib>:"CTRE_Phoenix_MotorControl_RefNumRegistryGet.vi"() -> ("PhoenixMotorControlDevRef"=w3:T7)  [unwired: 10 in, 1 out]
  n19 = for {
    tunnel: [w51] -> _ mode=indexing
    tunnel: w6 -> [w52]
    tunnel: w4 -> [w51] mode=indexing
    shift-right: [w44] -> _
    shift-left: _ -> [_]
    shift-right: [w43] -> _
    shift-left: _ -> [_]
    tunnel: w3 -> [w22]
    tunnel: w1 -> [w21]
    n20 = Unbundle By Name(w51) -> ("Action"=w47:T12, "Effort"=w55:dbl, "Duration"=w50:dbl, "Encoder"=w54:dbl, "Condition"=w53:bool)
    n21 = Multiply(x=w50, y=100.0) -> (x*y=w48:dbl)
    n22 = case shown="\"Left Switch\"" w47 {
      tunnel: w55 -> [_ _ _ w125 _ _]
      tunnel: w54 -> [_ _ _ w124 _ _]
      tunnel: w53 -> [_ _ _ _ _ _]
      tunnel: w52 -> [w60 _ w95 _ w161 w195]
      tunnel: w48 -> [_ _ _ _ _ _]
      tunnel: w22 -> [w59 _ w92 _ w159 w193]
      tunnel: w21 -> [w58 _ w93 _ w158 w192]
      tunnel: [w57 _ w91 _ w157 w191] -> w20
      tunnel: [w56 _ w90 _ w156 w190] -> w19
      frame "Nothing" {
        n23 = String Subset(string=w60, offset (0)=1, length (rest)=2 ("length (rest)")) -> (substring=w61:string)
        n24 = case shown="\"L\"" w61 {
          tunnel: w59 -> [w66 w80]
          tunnel: w58 -> [w67 w79]
          tunnel: [w65 w78] -> w57
          tunnel: [w64 w77] -> w56
          frame "R" {
            w68 = refnum<class "MotionProfiles.lvclass"> refnum ("MotionProfiles.lvclass")
            n25 = call "MotionProfiles_Init.vi"("Wheel_Diameter (in)"=6.0, "MP_Frame_Rate_(ms)"=5, "Encoder_CPR_4x"=4096.0, "CSV File Path"=path "/home/lvuser/leftdrive.csv", "PhoenixMotorControlDevRef"=w66, "MotionProfiles in"=w68) -> ("MotionProfiles out"=w65:refnum<class "MotionProfiles.lvclass">)  [unwired: 4 in, 1 out]
            n26 = call "MotionProfiles_Init.vi"("Wheel_Diameter (in)"=6.0, "MP_Frame_Rate_(ms)"=5, "Encoder_CPR_4x"=4096.0, "CSV File Path"=path "/home/lvuser/rightdrive.csv", "PhoenixMotorControlDevRef"=w67, "MotionProfiles in"=w68) -> ("MotionProfiles out"=w64:refnum<class "MotionProfiles.lvclass">)  [unwired: 4 in, 1 out]
          }
          frame "L" {
            w85 = refnum<class "MotionProfiles.lvclass"> refnum ("MotionProfiles.lvclass")
            n27 = call "MotionProfiles_Init.vi"("Wheel_Diameter (in)"=6.0, "MP_Frame_Rate_(ms)"=5, "Encoder_CPR_4x"=4096.0, "CSV File Path"=path "/home/lvuser/leftmp.csv", "PhoenixMotorControlDevRef"=w80, "MotionProfiles in"=w85) -> ("MotionProfiles out"=w78:refnum<class "MotionProfiles.lvclass">)  [unwired: 4 in, 1 out]
            n28 = call "MotionProfiles_Init.vi"("Wheel_Diameter (in)"=6.0, "MP_Frame_Rate_(ms)"=5, "Encoder_CPR_4x"=4096.0, "CSV File Path"=path "/home/lvuser/rightmp.csv", "PhoenixMotorControlDevRef"=w79, "MotionProfiles in"=w85) -> ("MotionProfiles out"=w77:refnum<class "MotionProfiles.lvclass">)  [unwired: 4 in, 1 out]
          }
        }
      }
      frame "Nothing" {
      }
      frame "Drive" {
        n29 = String Subset(string=w95, offset (0)=1, length (rest)=2 ("length (rest)")) -> (substring=w94:string)
        n30 = case shown="\"R\"" w94 {
          tunnel: w93 -> [w101 w114]
          tunnel: w92 -> [w100 w113]
          tunnel: [w99 w112] -> w91
          tunnel: [w98 w111] -> w90
          frame "R" {
            w106 = refnum<class "MotionProfiles.lvclass"> refnum ("MotionProfiles.lvclass")
            n31 = call "MotionProfiles_Init.vi"("Wheel_Diameter (in)"=6.0, "MP_Frame_Rate_(ms)"=5, "Encoder_CPR_4x"=4096.0, "CSV File Path"=path "/home/lvuser/leftmp.csv", "PhoenixMotorControlDevRef"=w100, "MotionProfiles in"=w106) -> ("MotionProfiles out"=w99:refnum<class "MotionProfiles.lvclass">)  [unwired: 4 in, 1 out]
            n32 = call "MotionProfiles_Init.vi"("Wheel_Diameter (in)"=6.0, "MP_Frame_Rate_(ms)"=5, "Encoder_CPR_4x"=4096.0, "CSV File Path"=path "/home/lvuser/rightmp.csv", "PhoenixMotorControlDevRef"=w101, "MotionProfiles in"=w106) -> ("MotionProfiles out"=w98:refnum<class "MotionProfiles.lvclass">)  [unwired: 4 in, 1 out]
          }
          frame "L" {
            w115 = refnum<class "MotionProfiles.lvclass"> refnum ("MotionProfiles.lvclass")
            n33 = call "MotionProfiles_Init.vi"("Wheel_Diameter (in)"=6.0, "MP_Frame_Rate_(ms)"=5, "Encoder_CPR_4x"=4096.0, "CSV File Path"=path "/home/lvuser/leftmp.csv", "PhoenixMotorControlDevRef"=w113, "MotionProfiles in"=w115) -> ("MotionProfiles out"=w112:refnum<class "MotionProfiles.lvclass">)  [unwired: 4 in, 1 out]
            n34 = call "MotionProfiles_Init.vi"("Wheel_Diameter (in)"=6.0, "MP_Frame_Rate_(ms)"=5, "Encoder_CPR_4x"=4096.0, "CSV File Path"=path "/home/lvuser/rightmp.csv", "PhoenixMotorControlDevRef"=w114, "MotionProfiles in"=w115) -> ("MotionProfiles out"=w111:refnum<class "MotionProfiles.lvclass">)  [unwired: 4 in, 1 out]
          }
        }
      }
      frame "Drive" {
        n35 = flat-sequence {
          tunnel: w125 -> [w127]
          tunnel: w124 -> [w126]
          frame #0 {
            n36 = while {
              tunnel: w127 -> [w130]
              tunnel: w126 -> [w128]
              stop <- w129 stop-if-true
              w143 = 0.75
              n37 = call "AutoDrive.vi"("Target"=w128, "Drive Effort"=w130) -> ()  [unwired: 10 in]
              n38 = global read "Global 2.vi" "LD Encoder Distance"() -> (w134:dbl)
              n39 = global read "Global 2.vi" "RD Encoder Distance"() -> (w135:dbl)
              n40 = Add(x=w135, y=w134) -> (x+y=w133:dbl)
              n41 = Divide(x=w133, y=2.0) -> (x/y=w131:dbl)
              n42 = Add(x=w128, y=w143) -> (x+y=w142:dbl)
              n43 = Subtract(x=w128, y=w143) -> (x-y=w141:dbl)
              n44 = In Range and Coerce(upper limit=w142, x=w131, lower limit=w141) -> (In Range?=w136:bool)  [unwired: 1 out]
              n45 = Not(x=w136) -> (.not. x?=w137:bool)
              n46 = call "Elapsed Time"("Time Target (s)"=0.25, "Reset"=w137) -> ("Present (s)"=→"Present (s) 2":dbl, "Elapsed Time (s)"=→"Elapsed Time (s) 2":dbl, "Time has Elapsed"=w129:bool)  [unwired: 10 in, 5 out]
              "Time has Elapsed 2" <- w129
            }
          }
          frame #1 {
            w144 = 0.0 ("Drive L")
            n47 = call <vilib>:"WPI_MotorControlRefNum Registry Get.vi"("refnum name"="Drive L0") -> ("error out"=w150:errorcluster, "MotorControlDevRef"=w151:T7)  [unwired: 9 in]
            n48 = call <vilib>:"WPI_MotorControlRefNum Registry Get.vi"("refnum name"="Drive L1") -> ("error out"=w154:errorcluster, "MotorControlDevRef"=w153:T7)  [unwired: 9 in]
            n49 = call <vilib>:"WPI_MotorControlRefNum Registry Get.vi"("refnum name"="Drive R0") -> ("error out"=w149:errorcluster, "MotorControlDevRef"=w145:T7)  [unwired: 9 in]
            n50 = call <vilib>:"WPI_MotorControlRefNum Registry Get.vi"("refnum name"="Drive R1") -> ("MotorControlDevRef"=w147:T7)  [unwired: 9 in, 1 out]
            n51 = call <vilib>:"WPI_MotorControlSetOutput.vi"("error in (no error)"=w150, "Output"=w144, "MotorControlDevRef"=w151) -> ()  [unwired: 6 in, 3 out]
            n52 = call <vilib>:"WPI_MotorControlSetOutput.vi"("error in (no error)"=w154, "Output"=w144, "MotorControlDevRef"=w153) -> ()  [unwired: 6 in, 3 out]
            n53 = call <vilib>:"WPI_MotorControlSetOutput.vi"("error in (no error)"=w149, "Output"=w144, "MotorControlDevRef"=w145) -> ()  [unwired: 6 in, 3 out]
            n54 = call <vilib>:"WPI_MotorControlSetOutput.vi"("Output"=w144, "MotorControlDevRef"=w147) -> ()  [unwired: 7 in, 3 out]
          }
        }
      }
      frame "Turn" {
        n55 = String Subset(string=w161, offset (0)=0, length (rest)=1 ("length (rest)")) -> (substring=w160:string)
        n56 = case shown="\"L\"" w160 {
          tunnel: w159 -> [w164 w180]
          tunnel: w158 -> [w165 w179]
          tunnel: [w167 w178] -> w157
          tunnel: [w166 w177] -> w156
          frame "R" {
            w168 = refnum<class "MotionProfiles.lvclass"> refnum ("MotionProfiles.lvclass")
            n57 = call "MotionProfiles_Init.vi"("Wheel_Diameter (in)"=6.0, "MP_Frame_Rate_(ms)"=5, "Encoder_CPR_4x"=4096.0, "CSV File Path"=path "/home/lvuser/leftmp.csv", "PhoenixMotorControlDevRef"=w164, "MotionProfiles in"=w168) -> ("MotionProfiles out"=w167:refnum<class "MotionProfiles.lvclass">)  [unwired: 4 in, 1 out]
            n58 = call "MotionProfiles_Init.vi"("Wheel_Diameter (in)"=6.0, "MP_Frame_Rate_(ms)"=5, "Encoder_CPR_4x"=4096.0, "CSV File Path"=path "/home/lvuser/rightmp.csv", "PhoenixMotorControlDevRef"=w165, "MotionProfiles in"=w168) -> ("MotionProfiles out"=w166:refnum<class "MotionProfiles.lvclass">)  [unwired: 4 in, 1 out]
          }
          frame "L" {
            w181 = refnum<class "MotionProfiles.lvclass"> refnum ("MotionProfiles.lvclass")
            n59 = call "MotionProfiles_Init.vi"("Wheel_Diameter (in)"=6.0, "MP_Frame_Rate_(ms)"=5, "Encoder_CPR_4x"=4096.0, "CSV File Path"=path "/home/lvuser/leftmp.csv", "PhoenixMotorControlDevRef"=w180, "MotionProfiles in"=w181) -> ("MotionProfiles out"=w178:refnum<class "MotionProfiles.lvclass">)  [unwired: 4 in, 1 out]
            n60 = call "MotionProfiles_Init.vi"("Wheel_Diameter (in)"=6.0, "MP_Frame_Rate_(ms)"=5, "Encoder_CPR_4x"=4096.0, "CSV File Path"=path "/home/lvuser/rightmp.csv", "PhoenixMotorControlDevRef"=w179, "MotionProfiles in"=w181) -> ("MotionProfiles out"=w177:refnum<class "MotionProfiles.lvclass">)  [unwired: 4 in, 1 out]
          }
        }
      }
      frame "Vision Correction" {
        n61 = String Subset(string=w195, offset (0)=0, length (rest)=1 ("length (rest)")) -> (substring=w194:string)
        n62 = case shown="\"R\"" w194 {
          tunnel: w193 -> [w200 w214]
          tunnel: w192 -> [w201 w213]
          tunnel: [w199 w212] -> w191
          tunnel: [w198 w211] -> w190
          frame "R" {
            w202 = refnum<class "MotionProfiles.lvclass"> refnum ("MotionProfiles.lvclass")
            n63 = call "MotionProfiles_Init.vi"("Wheel_Diameter (in)"=6.0, "MP_Frame_Rate_(ms)"=5, "Encoder_CPR_4x"=4096.0, "CSV File Path"=path "/home/lvuser/leftmp.csv", "PhoenixMotorControlDevRef"=w200, "MotionProfiles in"=w202) -> ("MotionProfiles out"=w199:refnum<class "MotionProfiles.lvclass">)  [unwired: 4 in, 1 out]
            n64 = call "MotionProfiles_Init.vi"("Wheel_Diameter (in)"=6.0, "MP_Frame_Rate_(ms)"=5, "Encoder_CPR_4x"=4096.0, "CSV File Path"=path "/home/lvuser/rightmp.csv", "PhoenixMotorControlDevRef"=w201, "MotionProfiles in"=w202) -> ("MotionProfiles out"=w198:refnum<class "MotionProfiles.lvclass">)  [unwired: 4 in, 1 out]
          }
          frame "L" {
            w215 = refnum<class "MotionProfiles.lvclass"> refnum ("MotionProfiles.lvclass")
            n65 = call "MotionProfiles_Init.vi"("Wheel_Diameter (in)"=6.0, "MP_Frame_Rate_(ms)"=5, "Encoder_CPR_4x"=4096.0, "CSV File Path"=path "/home/lvuser/leftmp.csv", "PhoenixMotorControlDevRef"=w214, "MotionProfiles in"=w215) -> ("MotionProfiles out"=w212:refnum<class "MotionProfiles.lvclass">)  [unwired: 4 in, 1 out]
            n66 = call "MotionProfiles_Init.vi"("Wheel_Diameter (in)"=6.0, "MP_Frame_Rate_(ms)"=5, "Encoder_CPR_4x"=4096.0, "CSV File Path"=path "/home/lvuser/rightmp.csv", "PhoenixMotorControlDevRef"=w213, "MotionProfiles in"=w215) -> ("MotionProfiles out"=w211:refnum<class "MotionProfiles.lvclass">)  [unwired: 4 in, 1 out]
          }
        }
      }
    }
    n67 = call "MotionProfiles_Control.vi"("MotionProfiles in"=w20) -> ("MotionProfiles out"=w46:refnum<class "MotionProfiles.lvclass">)  [unwired: 9 in, 1 out]
    n68 = call "MotionProfiles_Control.vi"("MotionProfiles in"=w19) -> ("MotionProfiles out"=w45:refnum<class "MotionProfiles.lvclass">)  [unwired: 9 in, 1 out]
    n69 = call "MotionProfiles_GetStatus.vi"("MotionProfiles in"=w46) -> ("MotionProfiles out"=w41:refnum<class "MotionProfiles.lvclass">, "MP_Class_Status"=w39:T13)  [unwired: 12 in, 1 out]
    n70 = call "MotionProfiles_GetStatus.vi"("MotionProfiles in"=w45) -> ("MotionProfiles out"=w42:refnum<class "MotionProfiles.lvclass">, "MP_Class_Status"=w40:T13)  [unwired: 12 in, 1 out]
    n71 = Unbundle By Name(w40) -> ("Motion Profile Status.Bottom Buffer Count"=→"Right Bottom Buf Count":i32, "Motion Profile Status.Is Underrun?"=→"Right Is Under Run":bool, "Set_Vel_(u/100ms)"=w35:i32, "Act_Vel_(u/100ms)"=w34:i32, "Set_Pos_(u)"=w33:i32, "Act_Pos(u)"=w32:i32, "Throtle"=→"Right Throttle":dbl)
    n72 = Unbundle By Name(w39) -> ("Motion Profile Status.Bottom Buffer Count"=→"Left Bottom Buf Count":i32, "Motion Profile Status.Is Underrun?"=→"Left Is Under Run":bool, "Set_Vel_(u/100ms)"=w29:i32, "Act_Vel_(u/100ms)"=w28:i32, "Set_Pos_(u)"=w27:i32, "Act_Pos(u)"=w26:i32, "Throtle"=→"Left Throttle":dbl)
    n73 = call "MotionProfiles_Start.vi"("MotionProfiles in"=w41) -> ("MotionProfiles out"=w44:refnum<class "MotionProfiles.lvclass">)  [unwired: 9 in, 1 out]
    n74 = call "MotionProfiles_Start.vi"("MotionProfiles in"=w42) -> ("MotionProfiles out"=w43:refnum<class "MotionProfiles.lvclass">)  [unwired: 9 in, 1 out]
    n75 = Bundle("Set_Vel_(u/100ms)"=w35, "Act_Vel_(u/100ms)"=w34, "Set_Pos_(u)"=w33, "Act_Pos(u)"=w32) -> (→"Right Motor":T1)  [unwired: 1 in]
    n76 = Bundle("Set_Vel_(u/100ms)"=w29, "Act_Vel_(u/100ms)"=w28, "Set_Pos_(u)"=w27, "Act_Pos(u)"=w26) -> (→"Left Motor":T1)  [unwired: 1 in]
  }
